vi "ELVIS III v1.0 Reserve AI.vi"(7 "Allow multiple opens?":bool, 8 "error in (no error)":errorcluster, 10 "AI Channel List":T2, 11 "myRIO FPGA Ref Out":T1) -> (0 "error out":errorcluster)   [LabVIEW 2021]
uses:
  <vilib>/myRIO/Common/Instrument Driver Framework/myRIO v1.0/AI/typedefs/AI Channels List.ctl
  <vilib>/myRIO/Common/Instrument Driver Framework/myRIO v1.0/AI/typedefs/AI Channels Enum.ctl
  <vilib>/myRIO/Common/Instrument Driver Framework/Utilities/typedefs/Generic FPGA Reference.ctl
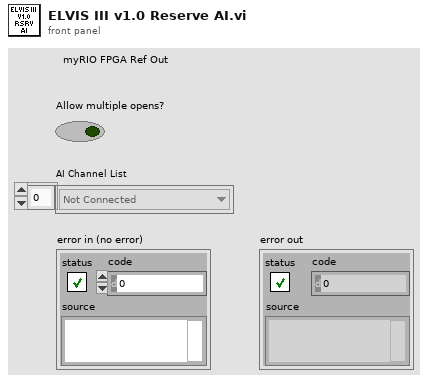
[diagram p1: front panel]
types:
  T1 = typedef "Generic FPGA Reference.ctl" = refnum<k20>
  T2 = typedef "AI Channels List.ctl" = T3[]
  T3 = typedef "AI Channels Enum.ctl" = enum16{"Not Connected", "AudioIn/Left", "AudioIn/Right", "C/AI0", "C/AI1", "A/AI0", "A/AI1", "A/AI2", "A/AI3", "A/AI4", "A/AI5", "A/AI6", "A/AI7", "B/AI0", "B/AI1", "B/AI2", "B/AI3", "B/AI4", "B/AI5", "B/AI6", "B/AI7", "AI/AI0", "AI/AI1", "AI/AI2", "AI/AI3", "A/AI0 (DIFF)", "A/AI1 (DIFF)", "A/AI2 (DIFF)", "A/AI3 (DIFF)", "B/AI0 (DIFF)", "B/AI1 (DIFF)", "B/AI2 (DIFF)", "B/AI3 (DIFF)"}
  T4 = typedef "ELVIS III v1.0 Channel Reservation List.ctl" = T5[]
  T5 = typedef "ELVIS III v1.0 Channel Reservation Info.ctl" = cluster{"Channel Name":string, "Connector":T6, "MutexIDs":u32[]}
  T6 = typedef "ELVIS III v1.0 Connector List.ctl" = enum32{"None", "ConnectorA", "ConnectorB"}
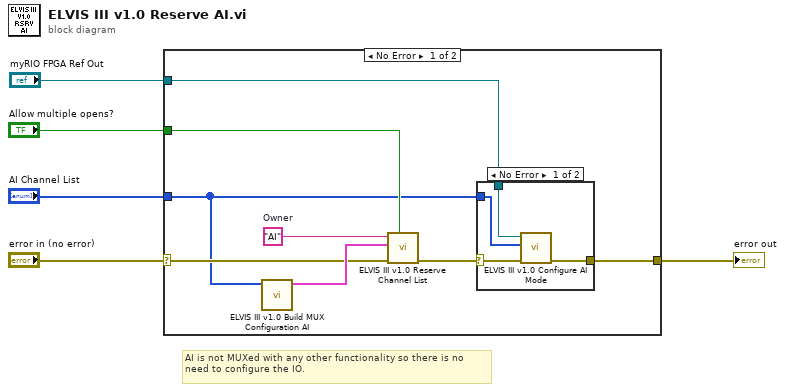
[diagram p0: block diagram]
diagram:
  # "AI is not MUXed with any other functionality so there is no need to configure the IO."
  n1 = case shown="No Error" "error in (no error)" {
    selector: "error in (no error)" -> [w11 w19]
    tunnel: "Allow multiple opens?" -> [w10 _]
    tunnel: "AI Channel List" -> [w6 _]
    tunnel: [w7 w19] -> w4
    tunnel: "myRIO FPGA Ref Out" -> [w8 _]
    frame No Error {
      w13 = "AI"  # Owner
      n2 = call <vilib>:"ELVIS III v1.0 Build MUX Configuration AI.vi"("AI Channels List"=w6) -> ("Channel Reservation Info"=w12:T4)  [unwired: 10 in]
      n3 = call <vilib>:"ELVIS III v1.0 Reserve Channel List.vi"("Allow multiple opens?"=w10, "error in (no error)"=w11, "Channel Reservation List"=w12, "Owner"=w13) -> ("error out"=w9:errorcluster)  [unwired: 7 in]
      n4 = case shown="No Error" w9 {
        selector: w9 -> [w17 w18]
        tunnel: w8 -> [w15 _]
        tunnel: [w16 w18] -> w7
        tunnel: w6 -> [w14 _]
        frame No Error {
          n5 = call <vilib>:"ELVIS III v1.0 Configure AI Mode.vi"("error in (no error)"=w17, "AI Channel List"=w14, "myRIO FPGA Ref Out"=w15) -> ("error out"=w16:errorcluster)  [unwired: 8 in]
        }
        frame Error {
        }
      }
    }
    frame Error {
      # "There is an incoming error so there is nothing to do."
    }
  }
  "error out" <- w4
